vi "Log Event.vi"(8 "error in":errorcluster, 10 "Event Data":T1, 11 "Report in":refnum<class "Report.lvclass">) -> (0 "error out":errorcluster, 3 "Report out":refnum<class "Report.lvclass">)   [LabVIEW 2023, in "Report.lvlib" / "Report.lvclass"]
uses:
  Report.lvclass
  Custom Controls/Event Data.ctl
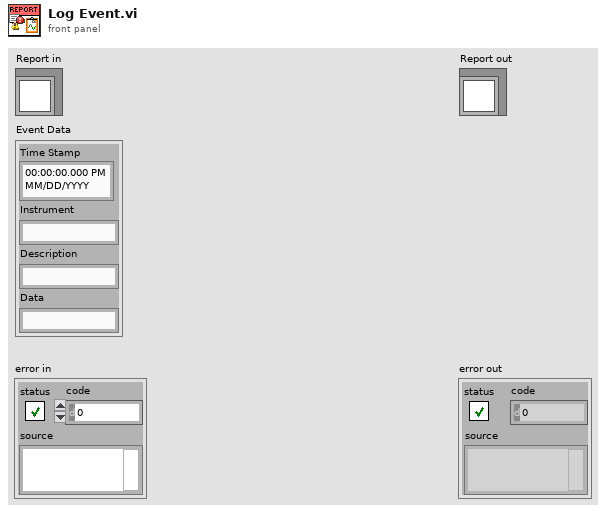
[diagram p1: front panel]
types:
  T1 = typedef "Report.lvlib/Report.lvclass/Event Data.ctl" = cluster{"Time Stamp":timestamp, "Instrument":string, "Description":string, "Data":string}
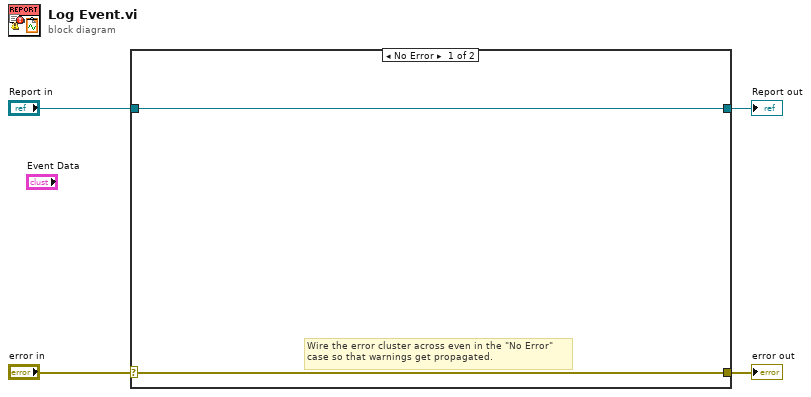
[diagram p0: block diagram]
diagram:
  n1 = case shown="No Error" "error in" {
    selector: "error in" -> [w5 w8]
    tunnel: [w5 w8] -> w3
    tunnel: [w6 w7] -> w1
    tunnel: "Report in" -> [w6 w7]
    frame No Error {
      # "Wire the error cluster across even in the \"No Error\"\ncase so that warnings get propagated."
    }
    frame Error {
    }
  }
  "error out" <- w3
  "Report out" <- w1
